vi "Transfer Group.Set Transceiver ID.vi"(10 "transceiver id":i32, 11 "Transfer Group in":refnum<class "Transfer Group.lvclass">) -> (3 "Transfer Group out":refnum<class "Transfer Group.lvclass">)   [LabVIEW 2017, in "DSF.Engine.lvlib" / "Transfer Group.lvclass"]
uses:
  Transfer Group.lvclass
  Transfer Group.lvclass/Transfer Group.ctl
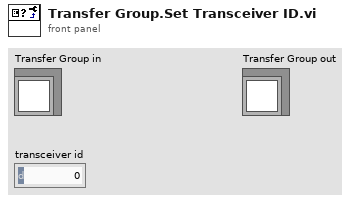
[diagram p1: front panel]
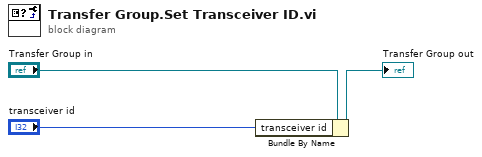
[diagram p0: block diagram]
diagram:
  n1 = Bundle By Name(cluster="Transfer Group in", "transceiver id"="transceiver id") -> (→"Transfer Group out":refnum<class "Transfer Group.lvclass">)
